vi "Control Panel.vi"(8 "error in (no error)":errorcluster, 11 "Power Meter in":refnum<class "Power Meter.lvclass">) -> (0 "error out":errorcluster, 3 "Power Meter out":refnum<class "Power Meter.lvclass">)   [LabVIEW 2012, in "Power Meter.lvclass"]
doc: "(Dynamic) A user-level application that simulates the physical front panel of the Instrument. Provide the user with buttons to manually control features of the instrument, and provide indicators of its current state."
uses:
  Power Meter.lvclass
  Newport 1830-C/Public/Filters.ctl
  Power Meter.lvclass/Power Meter.ctl
  Global/GPIB Numbers.vi
  Utility Classes/Readable/Readable.lvclass
  Utility Classes/Instrument/Instrument.lvclass
panel:
  out "connected?":bool
  out "Actual Power":dbl
  in  "Measured Power":dbl
  in  "Convert Power":bool
  out "Initialized?":bool
  in  "Filter":T1=1 items=["Orange"=1, "Green"=2, "Yellow"=3]
  out "Power":string
  in  "Time between Reads (ms)":i32=200
  in  "Read Continuous":bool
  in  "Averaging Time (s)":dbl=0.5
  in  "Averaging":bool
  out "Units":u16(ring)=1 items=["W"=1, "dB"=2, "dBm"=3, "REL"=4]
  out "AVG":u16(ring)=2 items=["Slow"=1, "Medium"=2, "Fast"=3]
  out "Run/Stop":u16(ring) items=["Stop", "Run"]
  out "ATTN":u16(ring) items=["Off", "On"]
  out "Local Lockout":u16(ring) items=["Off", "On"]
  out "Zero":u16(ring) items=["Off", "On"]
  out "Beeper":u16(ring) items=["Off", "On"]
  out "Backlight":u16(ring) items=["Off", "Low", "High"]
  out "Range":u16(ring) items=["Auto", "Highest Sensitivity", "30uW", "300uW", "3mW", "30mW", "300mW", "3W", "Lowest Sensitivity"]
  in  "Run/Stop set":u32(ring)=1 items=["Stop", "Run"]
  in  "ATTN set":u32(ring) items=["Off", "On"]
  in  "BKLT set":u32(ring)=1 items=["Off", "Low", "High"]
  in  "Range set":u32(ring) items=["Auto", "Highest Sensitivity", "30uW", "300uW", "3mW", "30mW", "300mW", "3W", "Lowest Sensitivity"]
  in  "Beeper set":u32(ring) items=["Off", "On"]
  in  "AVG set":u32(ring)=2 items=["Slow"=1, "Medium"=2, "Fast"=3]
  in  "Units set":u32(ring)=1 items=["W"=1, "dB"=2, "mdB"=3, "REL"=4]
  in  "Zero set":u32(ring) items=["Off", "On"]
  in  "Local set":u32(ring) items=["Off", "On"]
  in  "Read Current Power":bool
  in  "Set":bool
  in  "Read to \nControl":bool
  in  "Read":bool
  in  "Wavelength Set":dbl[unit]
  out "Wavelength":dbl[unit]
  in  "Copy actual to set":bool
  in  "Populate fields with member data":bool
  in  "stop":bool
  # "With \nAttn\nOn"
  # "Convert Measured Power"
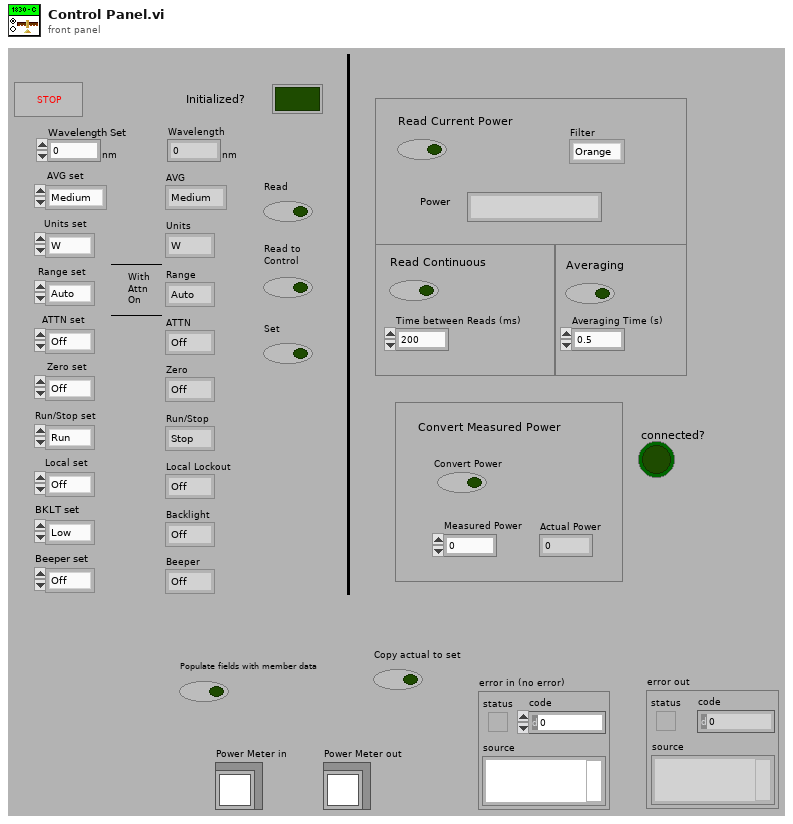
[diagram p1: front panel]
types:
  T1 = typedef "Filters.ctl" = u16
  T2 = enum8{"Enabled", "Disabled", "Disabled and Grayed Out"}
  T3 = typedef "GPIB Type Def.ctl" = cluster{"Name":string, "bus":dbl, "GPIB":dbl, "GPIB as string":string, "byte":i32, "VISA Resource Name":refnum<visa-resource-name>}
  T4 = typedef "Readable.lvclass/X array.ctl" = T5[]
  T5 = typedef "Readable.lvclass/X.ctl" = dbl
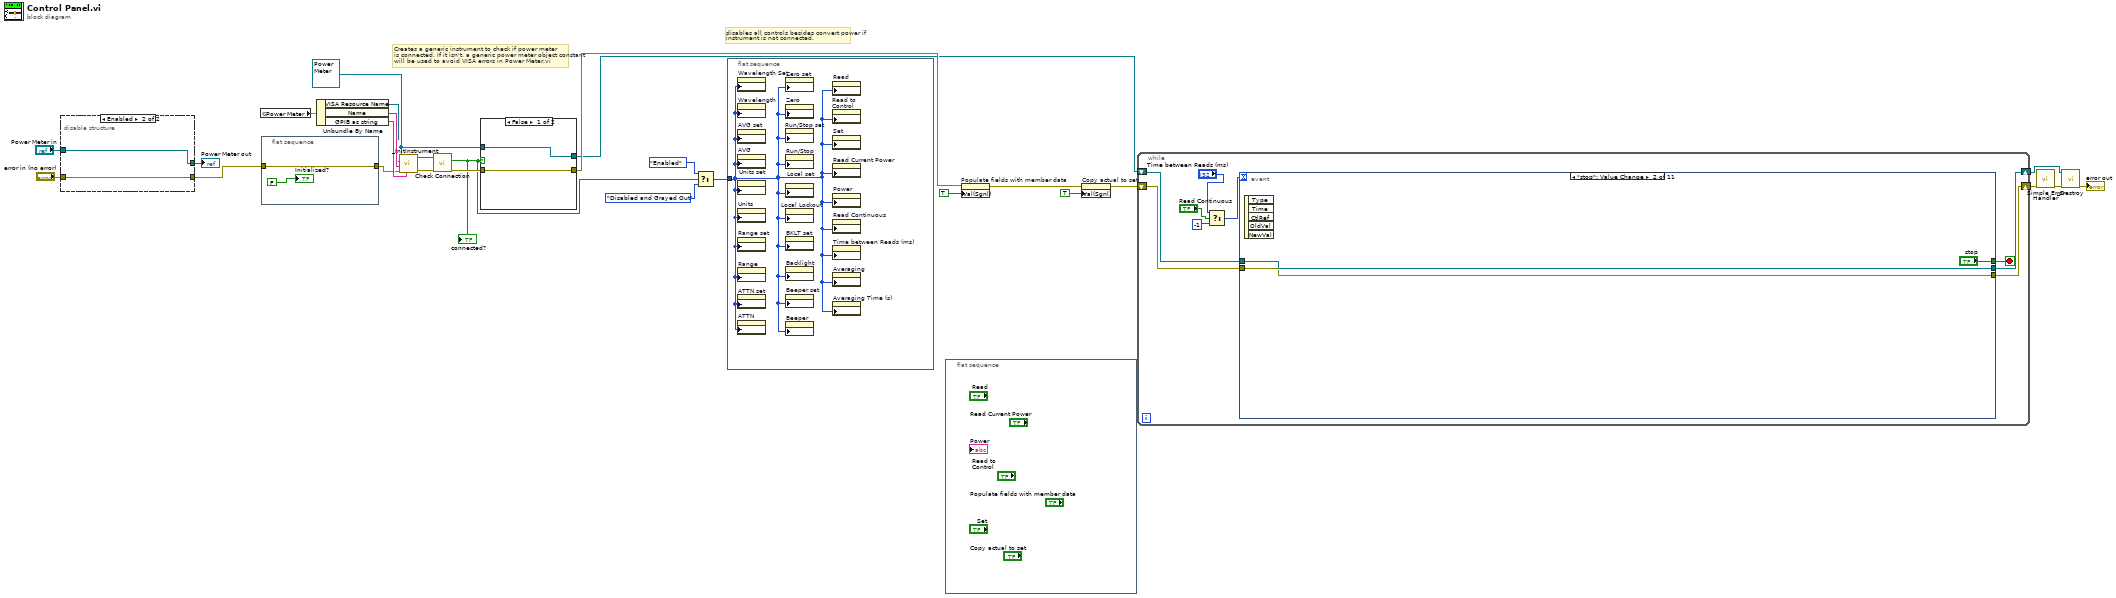
[diagram p0: block diagram]
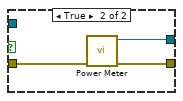
[diagram p2: hidden frame]
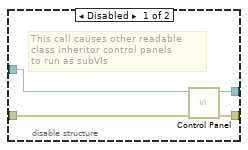
[diagram p3: hidden frame]
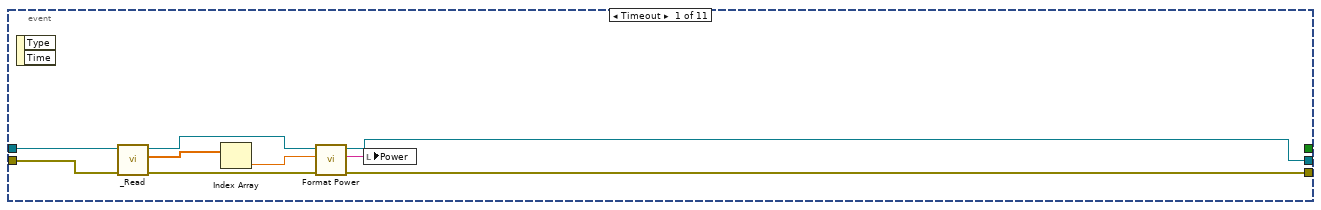
[diagram p4: hidden frame]
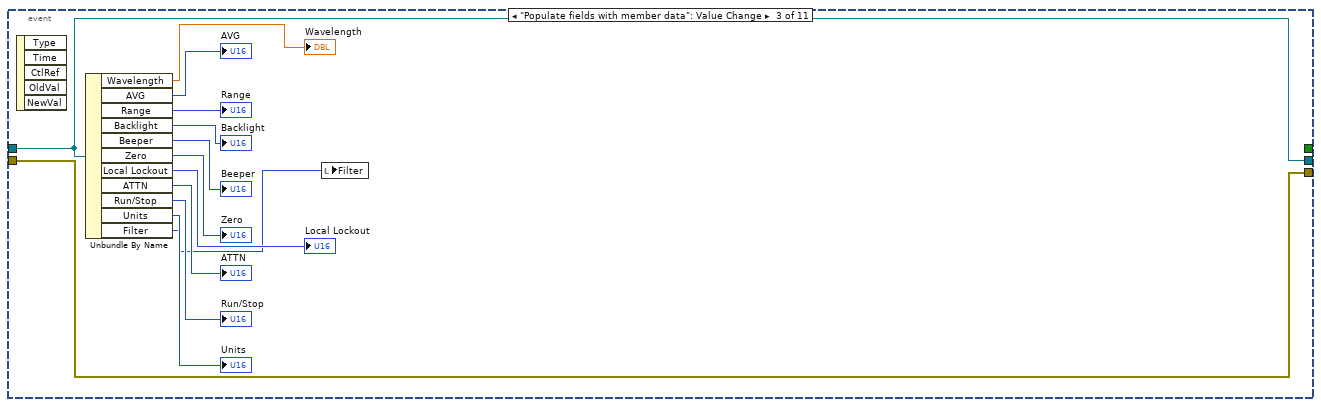
[diagram p5: hidden frame]
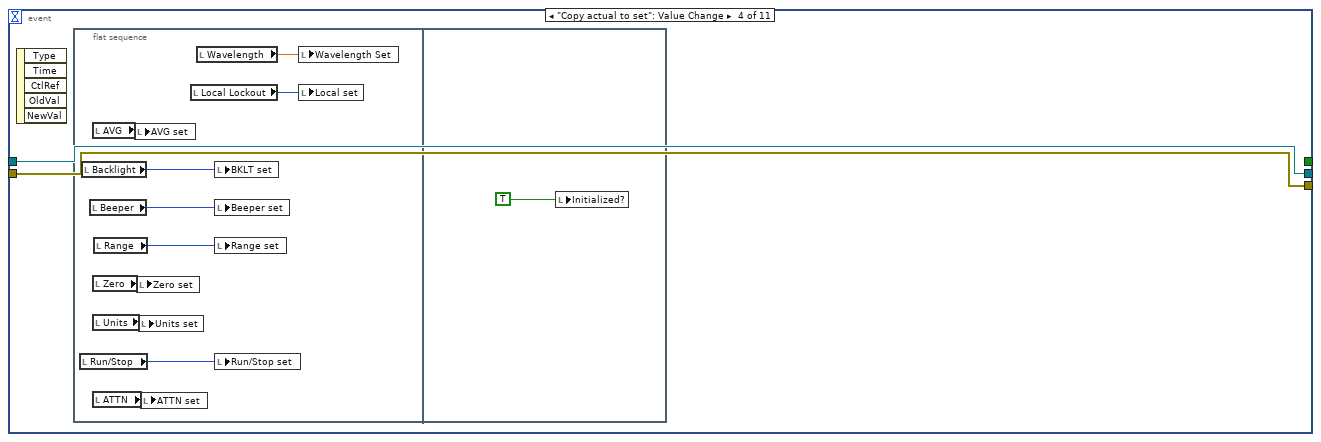
[diagram p6: hidden frame]
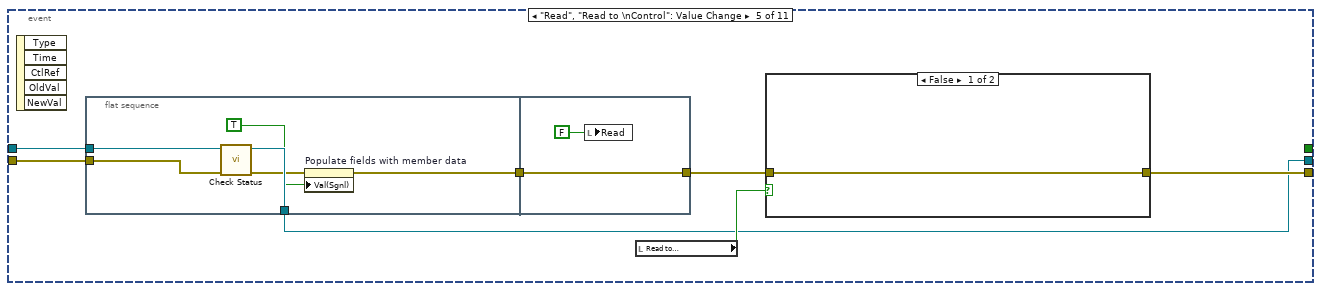
[diagram p7: hidden frame]
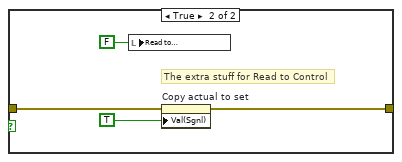
[diagram p8: hidden frame]
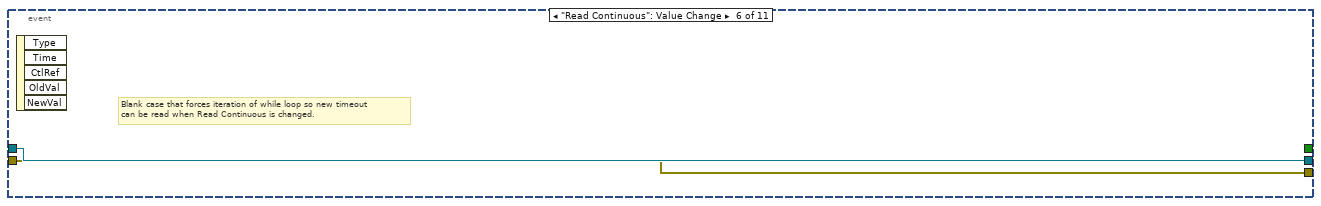
[diagram p9: hidden frame]
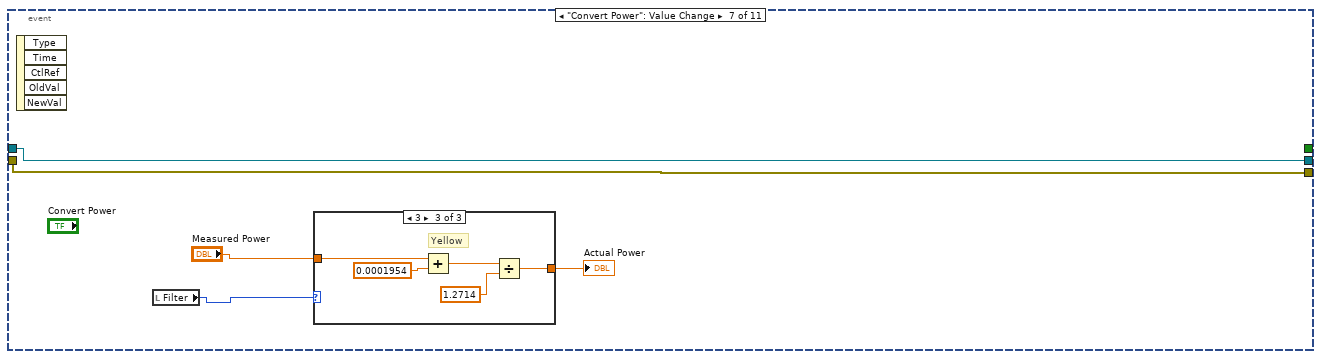
[diagram p10: hidden frame]
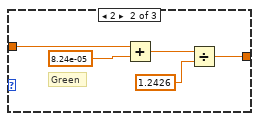
[diagram p12: hidden frame]
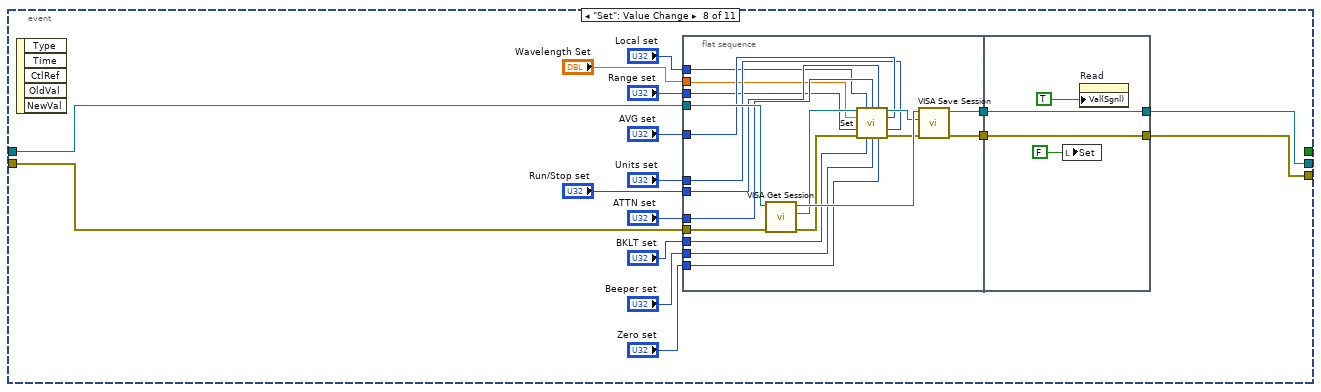
[diagram p13: hidden frame]
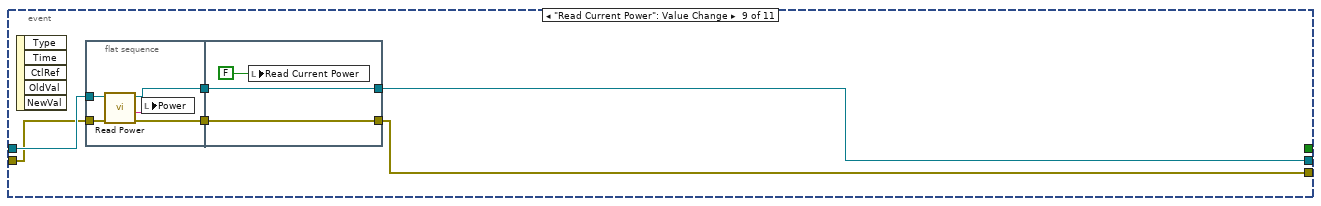
[diagram p14: hidden frame]
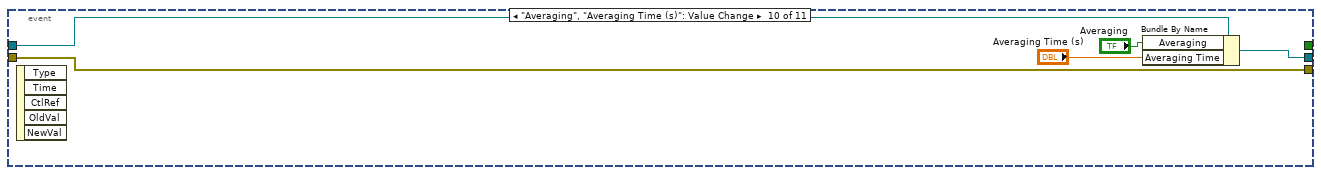
[diagram p15: hidden frame]
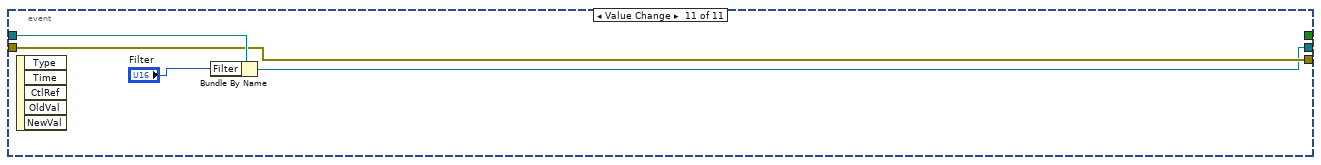
[diagram p16: hidden frame]
diagram:
  w1 = refnum<class "Power Meter.lvclass"> refnum ("Power Meter out")
  # "Creates a generic instrument to check if power meter\nis connected. If it isn't, a generic power meter object constant\nwill be used to avoid VISA errors in Power Meter.vi"
  # "disables all controls besides convert power if\ninstrument is not connected."
  n1 = disable-structure shown="Enabled" {
    disable-tunnel: "error in (no error)" -> [w31 w32]
    disable-tunnel: "Power Meter in" -> [w30 w33]
    disable-tunnel: [w29 w33] -> w25
    disable-tunnel: [w28 w32] -> w16
    frame Disabled {
      # "This call causes other readable\nclass inheritor control panels\nto run as subVIs"
      n2 = call-parent "Control Panel.vi"("error in (no error)"=w31, "Instrument in"=w30) -> ("error out"=w28:errorcluster, "Instrument out"=w29:refnum<class "Power Meter.lvclass">)  [unwired: 8 in]
    }
    frame Enabled {
    }
  }
  "Power Meter out" <- w25
  n3 = global read "GPIB Numbers.vi" "Power Meter"() -> (w12:T3)
  n4 = flat-sequence {
    tunnel: w16 -> [w34]
    tunnel: [w34] -> w8
    frame #0 {
      "Initialized?" <- FALSE
    }
  }
  n5 = Unbundle By Name(w12) -> ("VISA Resource Name"=w9:refnum<visa-resource-name>, "Name"=w10:string, "GPIB as string"=w11:string)
  n6 = call-dynamic "_InitInstrument.vi"("GPIB as string"=w11, "error in (no error)"=w8, "Name"=w10, "VISA Resource Name"=w9, "Instrument in"=w1) -> ("error out"=w7:errorcluster, "Instrument out"=w6:refnum<class "Power Meter.lvclass">)  [unwired: 1 in, 4 out]
  n7 = call "Check Connection.vi"("error in (no error)"=w7, "Instrument.lvclass in"=w6) -> ("error out"=w5:errorcluster, "connected?"=w4:bool)  [unwired: 7 in, 1 out]
  "connected?" <- w4
  n8 = case shown="False" w4 {
    tunnel: w5 -> [w37 w40]
    tunnel: [w37 w39] -> w3
    tunnel: [w36 w38] -> w2
    tunnel: w1 -> [w36 _]
    frame False {
    }
    frame True {
      n9 = call "Power Meter.vi"("error in (no error)"=w40) -> ("error out"=w39:errorcluster, "Power Meter out"=w38:refnum<class "Power Meter.lvclass">)  [unwired: 9 in]
    }
  }
  n10 = Select(t=T2."Enabled" ("Disabled"), s=w4, f=T2."Disabled and Grayed Out" ("Disabled")) -> (s? t:f=w13:T2)
  n11 = flat-sequence {
    tunnel: w13 -> [w41]
    frame #0 {
      n12 = property on="Wavelength Set" class="DigNum (strict)"("DisabledEnum"=w41) -> ()  [unwired: 2 in, 2 out]
      n13 = property on="Wavelength" class="DigNum (strict)"("DisabledEnum"=w41) -> ()  [unwired: 2 in, 2 out]
      n14 = property on="AVG set" class="Ring (strict)"("DisabledEnum"=w41) -> ()  [unwired: 2 in, 2 out]
      n15 = property on="AVG" class="Ring (strict)"("DisabledEnum"=w41) -> ()  [unwired: 2 in, 2 out]
      n16 = property on="Units set" class="Ring (strict)"("DisabledEnum"=w41) -> ()  [unwired: 2 in, 2 out]
      n17 = property on="Units" class="Ring (strict)"("DisabledEnum"=w41) -> ()  [unwired: 2 in, 2 out]
      n18 = property on="Range set" class="Ring (strict)"("DisabledEnum"=w41) -> ()  [unwired: 2 in, 2 out]
      n19 = property on="Range" class="Ring (strict)"("DisabledEnum"=w41) -> ()  [unwired: 2 in, 2 out]
      n20 = property on="ATTN set" class="Ring (strict)"("DisabledEnum"=w41) -> ()  [unwired: 2 in, 2 out]
      n21 = property on="ATTN" class="Ring (strict)"("DisabledEnum"=w41) -> ()  [unwired: 2 in, 2 out]
      n22 = property on="Zero set" class="Ring (strict)"("DisabledEnum"=w41) -> ()  [unwired: 2 in, 2 out]
      n23 = property on="Zero" class="Ring (strict)"("DisabledEnum"=w41) -> ()  [unwired: 2 in, 2 out]
      n24 = property on="Run/Stop set" class="Ring (strict)"("DisabledEnum"=w41) -> ()  [unwired: 2 in, 2 out]
      n25 = property on="Run/Stop" class="Ring (strict)"("DisabledEnum"=w41) -> ()  [unwired: 2 in, 2 out]
      n26 = property on="Local set" class="Ring (strict)"("DisabledEnum"=w41) -> ()  [unwired: 2 in, 2 out]
      n27 = property on="Local Lockout" class="Ring (strict)"("DisabledEnum"=w41) -> ()  [unwired: 2 in, 2 out]
      n28 = property on="BKLT set" class="Ring (strict)"("DisabledEnum"=w41) -> ()  [unwired: 2 in, 2 out]
      n29 = property on="Backlight" class="Ring (strict)"("DisabledEnum"=w41) -> ()  [unwired: 2 in, 2 out]
      n30 = property on="Beeper set" class="Ring (strict)"("DisabledEnum"=w41) -> ()  [unwired: 2 in, 2 out]
      n31 = property on="Beeper" class="Ring (strict)"("DisabledEnum"=w41) -> ()  [unwired: 2 in, 2 out]
      n32 = property on="Read" class="Bool (strict)"("DisabledEnum"=w41) -> ()  [unwired: 2 in, 2 out]
      n33 = property on="Read to \nControl" class="Bool (strict)"("DisabledEnum"=w41) -> ()  [unwired: 2 in, 2 out]
      n34 = property on="Set" class="Bool (strict)"("DisabledEnum"=w41) -> ()  [unwired: 2 in, 2 out]
      n35 = property on="Read Current Power" class="Bool (strict)"("DisabledEnum"=w41) -> ()  [unwired: 2 in, 2 out]
      n36 = property on="Power" class="Str"("DisabledEnum"=w41) -> ()  [unwired: 2 in, 2 out]
      n37 = property on="Read Continuous" class="Bool (strict)"("DisabledEnum"=w41) -> ()  [unwired: 2 in, 2 out]
      n38 = property on="Time between Reads (ms)" class="DigNum (strict)"("DisabledEnum"=w41) -> ()  [unwired: 2 in, 2 out]
      n39 = property on="Averaging" class="Bool (strict)"("DisabledEnum"=w41) -> ()  [unwired: 2 in, 2 out]
      n40 = property on="Averaging Time (s)" class="DigNum (strict)"("DisabledEnum"=w41) -> ()  [unwired: 2 in, 2 out]
    }
  }
  n41 = flat-sequence {
    frame #0 {
    }
  }
  n42 = property on="Populate fields with member data" class="Bool (strict)"(error in=w3, "Val(Sgnl)"=TRUE ("Value (Signaling)")) -> (error out=w22:errorcluster)  [unwired: 1 in, 1 out]
  n43 = property on="Copy actual to set" class="Bool (strict)"(error in=w22, "Val(Sgnl)"=TRUE ("Value (Signaling)")) -> (error out=w21:errorcluster)  [unwired: 1 in, 1 out]
  n44 = while {
    shift-right: [w47] -> w20
    shift-left: w2 -> [w49]
    shift-right: [w46] -> w19
    shift-left: w21 -> [w48]
    stop <- w50 stop-if-true
    n45 = Select(t="Time between Reads (ms)", s="Read Continuous", f=-1) -> (s? t:f=w43:i32)
    n46 = event shown="[1] \"stop\": Value Change" {
      selector: _ -> [_ _ _ _ _ _ _ _ _ _ _]
      dyn-events: _ -> [_ _ _ _ _ _ _ _ _ _ _]
      timeout: w43 -> [_ _ _ _ _ _ _ _ _ _ _]
      tunnel: [_ "stop" _ _ _ _ _ _ _ _ _] -> w50
      tunnel: [w51 w61 w74 w77 w89 w110 w115 w138 w167 w183 w185] -> w47
      tunnel: w49 -> [w59 w61 w74 w77 w95 w110 w115 w141 w171 w184 w188]
      tunnel: [w52 w60 w73 w76 w90 w109 w114 w137 w166 w182 w186] -> w46
      tunnel: w48 -> [w58 w60 w73 w76 w94 w109 w114 w139 w169 w182 w186]
      event Timeout {
        n47 = event-data() -> ()  [unwired: 1 in, 2 out]
        n48 = call-dynamic "_Read.vi"("error in (no error)"=w58, "Power Meter in"=w59) -> ("error out"=w56:errorcluster, "X array"=w55:T4, "Power Meter out"=w57:refnum<class "Power Meter.lvclass">)  [unwired: 7 in]
        n49 = Index Array(array=w55) -> (element=w54:T5)  [unwired: 1 in]
        n50 = call "Format Power.vi"("error in"=w56, "Power"=w54, "Power Meter.lvclass In"=w57) -> ("error out"=w52:errorcluster, "Formatted Power"=w53:string, "Power Meter.lvclass Out"=w51:refnum<class "Power Meter.lvclass">)  [unwired: 6 in]
        n51 = local write "Power"(w53) -> ()
      }
      event "stop": Value Change {
        n52 = event-data() -> ()  [unwired: 1 in, 5 out]
      }
      event "Populate fields with member data": Value Change {
        n53 = event-data() -> ()  [unwired: 1 in, 5 out]
        n54 = Unbundle By Name(w74) -> ("Wavelength"=→"Wavelength":dbl[unit], "AVG"=→"AVG":u16, "Range"=→"Range":u16, "Backlight"=→"Backlight":u16, "Beeper"=→"Beeper":u16, "Zero"=→"Zero":u16, "Local Lockout"=→"Local Lockout":u16, "ATTN"=→"ATTN":u16, "Run/Stop"=→"Run/Stop":u16, "Units"=→"Units":u16, "Filter"=w63:T1)
        n55 = local write "Filter"(w63) -> ()
      }
      event "Copy actual to set": Value Change {
        n56 = event-data() -> ()  [unwired: 1 in, 5 out]
        n57 = flat-sequence {
          frame #0 {
            n58 = local read "Run/Stop"() -> (w81:u16)
            n59 = local read "Backlight"() -> (w85:u16)
            n60 = local read "Beeper"() -> (w84:u16)
            n61 = local read "AVG"() -> (w86:u16)
            n62 = local read "Zero"() -> (w78:u16)
            n63 = local read "Units"() -> (w80:u16)
            n64 = local read "ATTN"() -> (w79:u16)
            n65 = local read "Range"() -> (w82:u16)
            n66 = local write "AVG set"(w86) -> ()
            n67 = local write "Zero set"(w78) -> ()
            n68 = local write "Units set"(w80) -> ()
            n69 = local write "ATTN set"(w79) -> ()
            n70 = local read "Local Lockout"() -> (w83:u16)
            n71 = local read "Wavelength"() -> (w87:dbl[unit])
            n72 = local write "BKLT set"(w85) -> ()
            n73 = local write "Beeper set"(w84) -> ()
            n74 = local write "Range set"(w82) -> ()
            n75 = local write "Run/Stop set"(w81) -> ()
            n76 = local write "Wavelength Set"(w87) -> ()
            n77 = local write "Local set"(w83) -> ()
          }
          frame #1 {
            n78 = local write "Initialized?"(TRUE ("Power\nMeter\nInitialized?")) -> ()
          }
        }
      }
      event "Read", "Read to \nControl": Value Change {
        n79 = event-data() -> ()  [unwired: 1 in, 5 out]
        n80 = flat-sequence {
          tunnel: w95 -> [w106]
          tunnel: w94 -> [w105]
          tunnel: [w102] -> w91
          tunnel: [w104] -> w89
          tunnel: [w107] -> w92
          tunnel: w91 -> [w107]
          frame #0 {
            n81 = call-dynamic "Check Status.vi"("error in (no error)"=w105, "Power Meter in"=w106) -> ("error out"=w103:errorcluster, "Power Meter out"=w104:refnum<class "Power Meter.lvclass">)  [unwired: 6 in, 2 out]
            n82 = property on="Populate fields with member data" class="Bool (strict)"(error in=w103, "Val(Sgnl)"=TRUE ("Value (Signaling)")) -> (error out=w102:errorcluster)  [unwired: 1 in, 1 out]
          }
          frame #1 {
            n83 = local write "Read"(FALSE ("Read")) -> ()
          }
        }
        n84 = local read "Read to \nControl"() -> (w93:bool)
        n85 = case shown="False" w93 {
          tunnel: w92 -> [w96 w98]
          tunnel: [w96 w97] -> w90
          frame False {
          }
          frame True {
            # "The extra stuff for Read to Control"
            n86 = local write "Read to \nControl"(FALSE ("Read")) -> ()
            n87 = property on="Copy actual to set" class="Bool (strict)"(error in=w98, "Val(Sgnl)"=TRUE ("Value (Signaling)")) -> (error out=w97:errorcluster)  [unwired: 1 in, 1 out]
          }
        }
      }
      event "Read Continuous": Value Change {
        # "Blank case that forces iteration of while loop so new timeout\ncan be read when Read Continuous is changed."
        n88 = event-data() -> ()  [unwired: 1 in, 5 out]
      }
      event "Convert Power": Value Change {
        n89 = event-data() -> ()  [unwired: 1 in, 5 out]
        n90 = local read "Filter"() -> (w111:T1)
        n91 = case shown="3" w111 {
          tunnel: "Measured Power" -> [w116 w118 w123]
          tunnel: [w116 w117 w122] -> w112
          frame 1, Default {
            # "Orange"
          }
          frame 2 {
            # "Green"
            n92 = Add(x=w118, y=8.24e-05) -> (x+y=w119:dbl)
            n93 = Divide(x=w119, y=1.2426) -> (x/y=w117:dbl)
          }
          frame 3 {
            # "Yellow"
            n94 = Add(x=w123, y=0.0001954) -> (x+y=w124:dbl)
            n95 = Divide(x=w124, y=1.2714) -> (x/y=w122:dbl)
          }
        }
        "Actual Power" <- w112
      }
      event "Set": Value Change {
        n96 = event-data() -> ()  [unwired: 1 in, 5 out]
        n97 = flat-sequence {
          tunnel: [w159] -> w142
          tunnel: w141 -> [w160]
          tunnel: [w157] -> w140
          tunnel: w139 -> [w158]
          tunnel: "AVG set" -> [w152]
          tunnel: "Units set" -> [w151]
          tunnel: "Run/Stop set" -> [w150]
          tunnel: "ATTN set" -> [w149]
          tunnel: "Local set" -> [w148]
          tunnel: "Wavelength Set" -> [w147]
          tunnel: "Range set" -> [w146]
          tunnel: "BKLT set" -> [w145]
          tunnel: "Beeper set" -> [w144]
          tunnel: "Zero set" -> [w143]
          tunnel: [w163] -> w138
          tunnel: w142 -> [w163]
          tunnel: [w162] -> w137
          tunnel: w140 -> [w162]
          frame #0 {
            n98 = call-dynamic "VISA Get Session.vi"("error in (no error)"=w158, "Instrument.lvclass in"=w160) -> ("error out"=w153:errorcluster, "VISA Resource Name"=w156:refnum<visa-resource-name>, "Instrument.lvclass out"=w161:refnum<class "Power Meter.lvclass">)  [unwired: 7 out]
            n99 = call "Set.vi"("VISA resource name"=w156, "Local Lockout (0:1)"=w148, "ATTN (0:1)"=w149, "Run/Stop (1:0)"=w150, "Wavelength (nnnn)"=w147, "AVG (1:3)"=w152, "Range (0-Auto,1:8)"=w146, "Units (1:4)"=w151, "error in (no error)"=w153, "Backlight (0:2)"=w145, "Beeper (0:1)"=w144, "Zero (0:1)"=w143) -> ("VISA resource name out"=w155:refnum<visa-resource-name>, "error out"=w154:errorcluster)  [unwired: 2 in]
            n100 = call-dynamic "VISA Save Session.vi"("error in (no error)"=w154, "VISA Resource Name"=w155, "Instrument.lvclass in"=w161) -> ("error out"=w157:errorcluster, "Instrument.lvclass out"=w159:refnum<class "Power Meter.lvclass">)  [unwired: 7 out]
          }
          frame #1 {
            n101 = local write "Set"(FALSE ("Set")) -> ()
            n102 = property on="Read" class="Bool (strict)"("Val(Sgnl)"=TRUE ("Value (Signaling)")) -> ()  [unwired: 2 in, 2 out]
          }
        }
      }
      event "Read Current Power": Value Change {
        n103 = event-data() -> ()  [unwired: 1 in, 5 out]
        n104 = flat-sequence {
          tunnel: w171 -> [w176]
          tunnel: [w172] -> w170
          tunnel: w169 -> [w175]
          tunnel: [w173] -> w168
          tunnel: [w178] -> w167
          tunnel: w170 -> [w178]
          tunnel: [w177] -> w166
          tunnel: w168 -> [w177]
          frame #0 {
            n105 = call "Read Power.vi"("error in (no error)"=w175, "Power Meter in"=w176) -> ("error out"=w173:errorcluster, "Current Power w/ Units"=w174:string, "Power Meter out"=w172:refnum<class "Power Meter.lvclass">)  [unwired: 6 in, 1 out]
            n106 = local write "Power"(w174) -> ()
          }
          frame #1 {
            n107 = local write "Read Current Power"(FALSE ("Read Current Value")) -> ()
          }
        }
      }
      event "Averaging", "Averaging Time (s)": Value Change {
        n108 = event-data() -> ()  [unwired: 1 in, 5 out]
        n109 = Bundle By Name(cluster=w184, "Averaging"="Averaging", "Averaging Time"="Averaging Time (s)") -> (w183:refnum<class "Power Meter.lvclass">)
      }
      event Value Change {
        n110 = event-data() -> ()  [unwired: 1 in, 5 out]
        n111 = Bundle By Name(cluster=w188, "Filter"="Filter") -> (w185:refnum<class "Power Meter.lvclass">)
      }
    }
  }
  n112 = call <vilib>:"Simple Error Handler.vi"("error in (no error)"=w19) -> ("error out"=w18:errorcluster)  [unwired: 1 in, 7 out]
  n113 = call-dynamic "_Destroy.vi"("error in (no error)"=w18, "Instrument in"=w20) -> ("error out"=→"error out":errorcluster)  [unwired: 9 out]
